vi "Refresh MCL and Buttons.vi"(8 "Error In":errorcluster) -> (0 "Error Out":errorcluster)   [LabVIEW 2023, in "Error Manager.lvlib"]
doc: "MCL = MultiColumn List\nMSEAR = \"Mark Selected Errors As Read\" button\nMAEAR = \"Mark All Errors As Read\" button"
uses:
  Error Manager.lvlib
  Queues/MHL Queue/Command (enum).ctl
  Queues/MHL Queue/MHL Queue.lvclass
panel:
  # "Input\nInputs to the VI"
  # "Development\nControls or indicators that are useful for development or testing, but which are not outputs of the VI."
  # "Output\nOutputs of the VI"
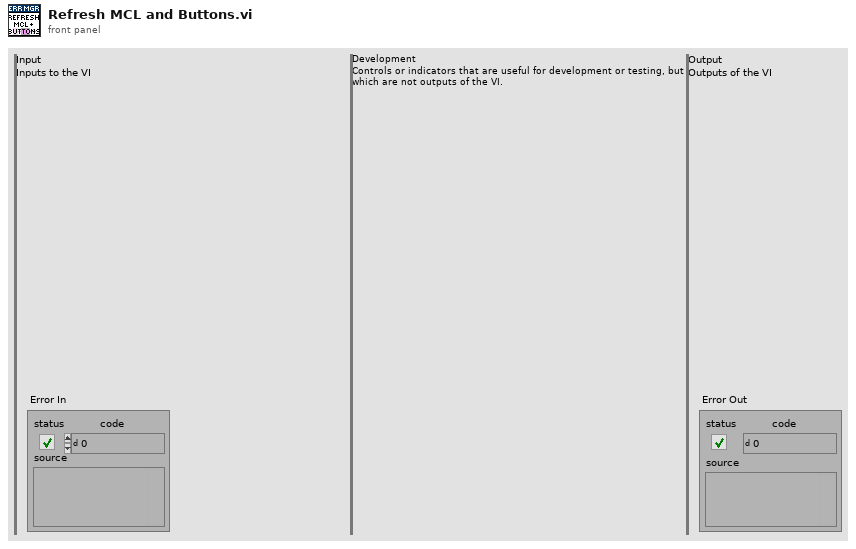
[diagram p1: front panel]
types:
  T1 = typedef "Error Manager.lvlib/MHL Queue.lvclass/Command (enum).ctl" = enum16{"Init Module", "Close Module", "Internal Error", "Create Error Log File", "Show Front Panel", "Handle Error", "Refresh MCL", "MCL Value Change", "Change Display Order", "One-Second Interval Expired", "Mark Selected Errors As Read", "Mark All Errors As Read", "Refresh Button State - MSEAR", "Refresh Button State - MAEAR"}
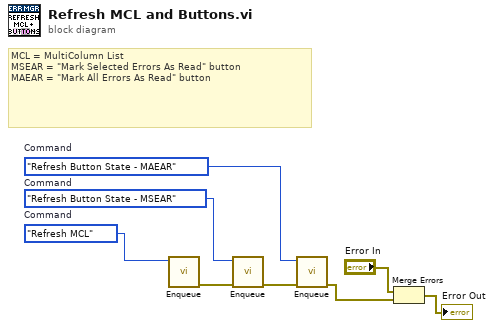
[diagram p0: block diagram]
diagram:
  w3 = Command_(enum)."Refresh Button State - MAEAR"  # Command
  w5 = Command_(enum)."Refresh Button State - MSEAR"  # Command
  w6 = Command_(enum)."Refresh MCL"  # Command
  # "MCL = MultiColumn List\nMSEAR = \"Mark Selected Errors As Read\" button\nMAEAR = \"Mark All Errors As Read\" button"
  n1 = call "Enqueue.vi"(11:w6) -> (0:w2:errorcluster)  [unwired: 10 in]
  n2 = call "Enqueue.vi"(8:w2, 11:w5) -> (0:w4:errorcluster)  [unwired: 9 in]
  n3 = call "Enqueue.vi"(8:w4, 11:w3) -> (0:w1:errorcluster)  [unwired: 9 in]
  n4 = Merge Errors("Error In", w1) -> (→"Error Out":errorcluster)
